vi "Filter Transaction By Coordinate Space.vi"(10 "Types In":T1[](array[typedef])=[enum."LVDT", enum."Actuator Command", enum."Displacement Command", enum."Load Cell", enum."Displacement", enum."Force", enum."Servo Error"], 11 "Coordinate Space":bool caption="Coord") -> (2 "Types Out":T1[](array[typedef])=[enum."LVDT"])   [LabVIEW 2009]
uses:
  Dataset Type.ctl
panel:
  in  "Cartesian Types":T1[](array[typedef])=[enum."Displacement Command", enum."Displacement", enum."Force"]
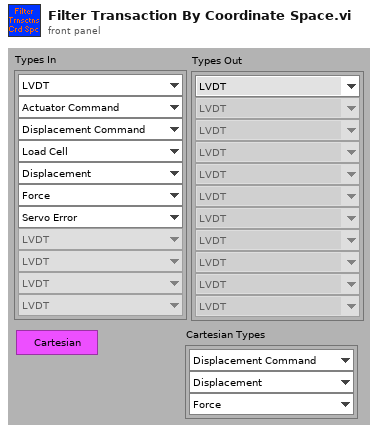
[diagram p1: front panel]
types:
  T1 = typedef "Dataset Type.ctl" = enum16{"LVDT", "Load Cell", "Actuator Command", "Servo Error", "Displacement Command", "Displacement", "Force"}
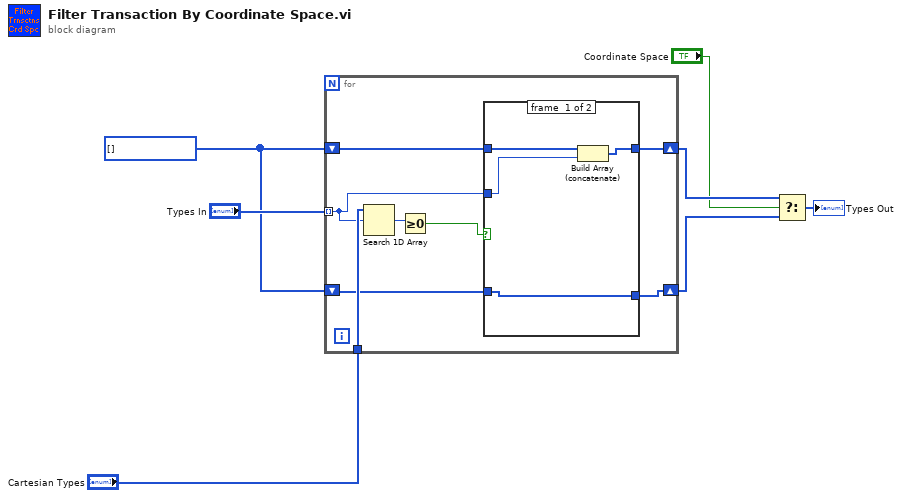
[diagram p0: block diagram]
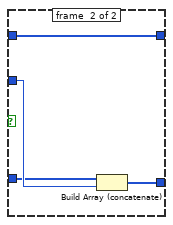
[diagram p2: hidden frame]
diagram:
  w1 = T1[] [] items=["LVDT", "Load Cell", "Actuator Command", "Servo Error", "Displacement Command", "Displacement", "Force"]
  n1 = for {
    tunnel: "Types In" -> [w12] mode=indexing
    tunnel: "Cartesian Types" -> [w15]
    shift-right: [w11] -> w4
    shift-left: w1 -> [w10]
    shift-right: [w9] -> w3
    shift-left: w1 -> [w8]
    n2 = Search 1D Array(1D array=w15, element=w12) -> (index of element=w14:i32)  [unwired: 1 in]
    n3 = Greater Or Equal To 0?(x=w14) -> (x >= 0?=w13:bool)
    n4 = case shown="False" w13 {
      tunnel: w12 -> [w19 w21]
      tunnel: [w18 w23] -> w11
      tunnel: w10 -> [w17 w23]
      tunnel: [w16 w22] -> w9
      tunnel: w8 -> [w16 w20]
      frame #0 {
        n5 = Build Array (concatenate)(w17, w19) -> (w18:T1[])
      }
      frame #1 {
        n6 = Build Array (concatenate)(w20, w21) -> (w22:T1[])
      }
    }
  }
  n7 = Select(t=w4, s="Coordinate Space", f=w3) -> (s? t:f=→"Types Out":T1[])
